vi "10進階題-數字持續加減.vi"() -> ()   [LabVIEW 2019]
panel:
  in  "Stop":bool
  out "N":i32
  in  "減1":bool
  in  "加1":bool
  # "每次按下Add及Dec，可以讓數字+1或-1。\n當持續按下超過1秒，N可快速增加或減少；超過3秒，速度更快。"
  # "復歸型按鍵"
  # "復歸型按鍵"
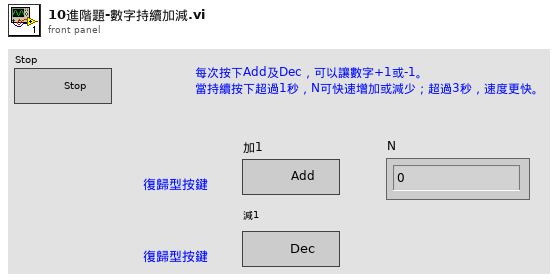
[diagram p1: front panel]
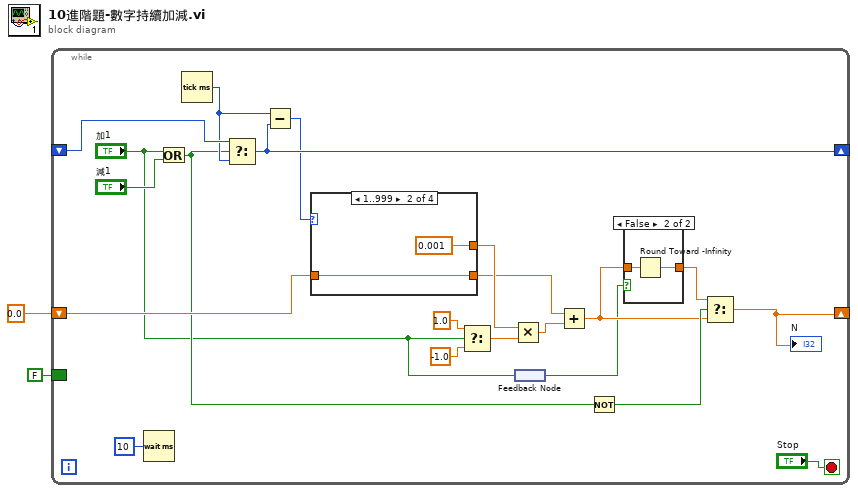
[diagram p0: block diagram]
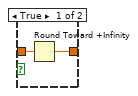
[diagram p2: hidden frame]
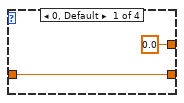
[diagram p3: hidden frame]
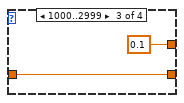
[diagram p4: hidden frame]
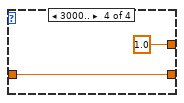
[diagram p5: hidden frame]
diagram:
  n1 = while {
    shift-right: [w21] -> _
    shift-left: _ -> [w23]
    shift-right: [w5] -> _
    shift-left: 0.0 -> [w17]
    border: FALSE ("加1") -> [_]
    stop <- "Stop" stop-if-true
    n2 = Wait (ms)(milliseconds to wait=u32 10) -> ()  [unwired: 1 out]
    n3 = Or(x="加1", y="減1") -> (x .or. y?=w9:bool)
    n4 = Tick Count (ms)() -> (millisecond timer value=w22:u32)
    n5 = Select(t=w23, s=w9, f=w22) -> (s? t:f=w21:u32)
    n6 = Subtract(x=w22, y=w21) -> (x-y=w19:u32)
    n7 = case shown="1..999" w19 {
      tunnel: [0.0 ("y") 0.001 ("y") 0.1 ("y") 1.0 ("y")] -> w12
      tunnel: w17 -> [w28 w30 w32 w34]
      tunnel: [w28 w30 w32 w34] -> w11
      frame 0, Default {
      }
      frame 1..999 {
      }
      frame 1000..2999 {
      }
      frame 3000.. {
      }
    }
    n8 = Select(t=1.0, s="加1", f=-1.0 ("t")) -> (s? t:f=w16:dbl)
    n9 = Multiply(x=w12, y=w16) -> (x*y=w10:dbl)
    n10 = feedback-in #1("加1") -> ()
    n11 = feedback #1() -> (w3:bool)
    n12 = Add(x=w11, y=w10) -> (x+y=w6:dbl)
    n13 = Not(x=w9) -> (.not. x?=w8:bool)
    n14 = case shown="False" w3 {
      tunnel: [w25 w27] -> w7
      tunnel: w6 -> [w24 w26]
      frame True {
        n15 = Round Toward +Infinity(x=w24) -> (ceil(x): smallest int >= x=w25:dbl)
      }
      frame False {
        n16 = Round Toward -Infinity(1:w26) -> (0:w27:dbl)
      }
    }
    n17 = Select(t=w7, s=w8, f=w6) -> (s? t:f=w5:dbl)
    "N" <- w5
  }
